vi "BundleByName.vi"() -> ()   [LabVIEW 2020]
panel:
  out "output cluster":T1
  in  "employee":T1={"Name"="Atul Ghumade", "Age"=29, "Salary"=100000, "Gender"=TRUE}
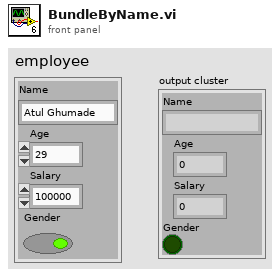
[diagram p1: front panel]
types:
  T1 = cluster{"Name":string, "Age":u8, "Salary":u32, "Gender":bool}
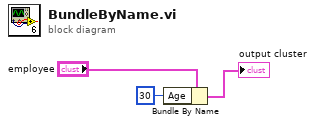
[diagram p0: block diagram]
diagram:
  n1 = Bundle By Name(cluster="employee", "Age"=u8 30) -> (→"output cluster":T1)
